vi "HFRR ADV v03.vi"() -> ()   [LabVIEW 2025] (continued)
          }
          n24 = Concatenate Strings(w97) -> (w93:string)
          n25 = local read "file path"() -> (w91:path)
          n26 = call <vilib>:"Write Characters To File.vi"("append to file? (new file:F)"=FALSE, "character string"=w93, "file path (dialog if empty)"=w91) -> ()  [unwired: 2 in, 1 out]
        }
      }
      n27 = local write "refresh flag"(FALSE ("refresh flag")) -> ()
      n28 = local write "Json End Flg"(w57) -> ()
      n29 = local write "Re-Initialise"(TRUE ("Re-Initialise")) -> ()
      n30 = local write "Upld AR 2"(TRUE ("Upld AR 2")) -> ()
      n31 = local write "Json St Flg"(w57) -> ()
      n32 = local write "FLAG 2"(0.0 ("FLAG 2")) -> ()
      n33 = local write "Lan flag"(0.0 ("Lan flag")) -> ()
      n34 = local write "Flag"(0.0 ("Flag")) -> ()
      n35 = local write "clk"(0.0 ("clk")) -> ()
      n36 = local write "COUNT"(0 ("COUNT")) -> ()
      n37 = case shown="True" "STOP" {
        frame False {
        }
        frame True {
          n38 = local write "STOP 3"(TRUE ("STOP")) -> ()
        }
      }
      n39 = local write "conststatus"(0.0 ("rpm value : 2")) -> ()
      "file path" <- path "C:/Windows/wndcm_pw_stdED hfrr.txt" ("file path")
      "FF buffer" <- dbl[] [] ("FF buffer")
    }
    frame #1 {
      n40 = Wait (ms)(milliseconds to wait=u32 1000) -> (millisecond timer value=w109:u32)
    }
    frame #2 {
      n41 = local read "Re-Initialise"() -> (w112:bool)
      n42 = case shown="True" w112 {
        frame False {
        }
        frame True {
          n43 = local write "Re-Initialise"(FALSE ("Re-Initialise")) -> ()
        }
      }
    }
  }
  n44 = local write "main tab sub"(enum32{"Page 1", "Page 2"}."Page 1" ("main tab sub")) -> ()
  n45 = local write "USERNAME"(w5) -> ()
  n46 = local write "USER ID"(w5) -> ()
  n47 = local write "Main Tab"(T1."HOME" ("Main Tab")) -> ()
  n48 = property on="Quit" class="Bool (strict)"("Value"=FALSE ("Quit")) -> (error out=w7:errorcluster)  [unwired: 2 in, 1 out]
  n49 = while {
    tunnel: w7 -> [_]
    stop <- w137 stop-if-true
    w128 = 1 ("y")
    # "New Adv Logics"
    n50 = local read "USERNAME"() -> (w134:string)
    n51 = local read "Sign In"() -> (w124:bool)
    n52 = local read "USER ID"() -> (w131:string)
    n53 = local read "Dashboard"() -> (w122:bool)
    n54 = local read "Imaging"() -> (w119:bool)
    n55 = local read "Test Setup"() -> (w123:bool)
    n56 = Wait (ms)(milliseconds to wait=u32 100) -> ()  [unwired: 1 out]
    n57 = case shown="True" w124 {
      selector: w124 -> [_ w164]
      frame False {
      }
      frame True {
        n58 = Not(x=w164) -> (.not. x?=w163:bool)
        n59 = local write "Sign In"(w163) -> ()
        n60 = local write "Main Tab"(T1."Test Setup" ("Main Tab")) -> ()
      }
    }
    n61 = call <vilib>:"Trim Whitespace.vi"("string"=w134) -> ("trimmed string"=w133:string)  [unwired: 1 in]
    n62 = call <vilib>:"Trim Whitespace.vi"("string"=w131) -> ("trimmed string"=w132:string)  [unwired: 1 in]
    n63 = case shown="True" w122 {
      selector: w122 -> [_ w158]
      frame False {
      }
      frame True {
        n64 = Not(x=w158) -> (.not. x?=w157:bool)
        n65 = local write "Dashboard"(w157) -> ()
        n66 = local write "Main Tab"(T1."Acquire" ("Main Tab")) -> ()
      }
    }
    n67 = String Length(string=w133) -> (length=w130:i32)
    n68 = String Length(string=w132) -> (length=w129:i32)
    n69 = case shown="True" w123 {
      selector: w123 -> [_ w161]
      frame False {
      }
      frame True {
        n70 = Not(x=w161) -> (.not. x?=w160:bool)
        n71 = local write "Test Setup"(w160) -> ()
        n72 = local write "Main Tab"(T1."HOME" ("Main Tab")) -> ()
      }
    }
    n73 = case shown="True" w119 {
      selector: w119 -> [_ w148]
      frame False {
      }
      frame True {
        n74 = Not(x=w148) -> (.not. x?=w147:bool)
        n75 = local write "Imaging"(w147) -> ()
        n76 = local write "Main Tab"(T1."Adv Scar" ("Main Tab")) -> ()
      }
    }
    n77 = local read "Main Tab"() -> (w135:T1)
    n78 = Greater?(x=w130, y=w128) -> (0:w127:bool)
    n79 = Greater?(x=w129, y=w128) -> (0:w126:bool)
    n80 = And(x=w127, y=w126) -> (x .and. y?=w125:bool)
    n81 = case shown="\"HOME\"" w135 {
      frame "HOME" {
        n82 = local write "main tab sub"(enum32{"Page 1", "Page 2"}."Page 1" ("main tab sub")) -> ()
      }
      frame Default {
        n83 = local write "main tab sub"(enum32{"Page 1", "Page 2"}."Page 2" ("main tab sub")) -> ()
      }
    }
    n84 = case shown="False" w125 {
      frame False {
        n85 = property on="Sign In" class="Bool (strict)"("DisabledEnum"=T11."Disabled" ("Disabled")) -> ()  [unwired: 2 in, 2 out]
      }
      frame True {
        n86 = property on="Sign In" class="Bool (strict)"("DisabledEnum"=T11."Enabled" ("Disabled")) -> ()  [unwired: 2 in, 2 out]
      }
    }
    n87 = local read "Report"() -> (w118:bool)
    n88 = local read "Button"() -> (w121:bool)
    n89 = case shown="True" w118 {
      selector: w118 -> [_ w145]
      frame False {
      }
      frame True {
        n90 = Not(x=w145) -> (.not. x?=w144:bool)
        n91 = local write "Report"(w144) -> ()
        n92 = local write "Main Tab"(T1."Adv Scar Report" ("Main Tab")) -> ()
      }
    }
    n93 = local read "Button 2"() -> (w120:bool)
    n94 = local read "Analysis"() -> (w117:bool)
    n95 = case shown="True" w121 {
      selector: w121 -> [_ w154]
      frame False {
      }
      frame True {
        n96 = Not(x=w154) -> (.not. x?=w153:bool)
        n97 = local write "Button"(w153) -> ()
        n98 = local write "Main Tab Display"(enum32{"Dashboard 1", "Dashboard 2"}."Dashboard 1" ("Main Tab Display")) -> ()
      }
    }
    n99 = case shown="True" w120 {
      selector: w120 -> [_ w152]
      frame False {
      }
      frame True {
        n100 = Not(x=w152) -> (.not. x?=w151:bool)
        n101 = local write "Button 2"(w151) -> ()
        n102 = local write "Main Tab Display"(enum32{"Dashboard 1", "Dashboard 2"}."Dashboard 2" ("Main Tab Display")) -> ()
      }
    }
    n103 = case shown="True" w117 {
      selector: w117 -> [_ w143]
      frame False {
      }
      frame True {
        n104 = Not(x=w143) -> (.not. x?=w141:bool)
        n105 = local write "Analysis"(w141) -> ()
        n106 = local write "Main Tab"(T1."Compare Files" ("Main Tab")) -> ()
      }
    }
    n107 = local read "About"() -> (w116:bool)
    n108 = case shown="True" w116 {
      selector: w116 -> [_ w140]
      frame False {
      }
      frame True {
        n109 = Not(x=w140) -> (.not. x?=w139:bool)
        n110 = local write "About"(w139) -> ()
        n111 = local write "Main Tab"(T1."About" ("Main Tab")) -> ()
      }
    }
    n112 = local read "Quit"() -> (w137:bool)
  }
  n113 = while {
    stop <- w173 stop-if-true
    n114 = local read "Image Path"() -> (w171:path)
    n115 = local read "Print 3"() -> (w175:bool)
    n116 = Equal?(x=w171, y=path "") -> (x = y?=w170:bool)
    n117 = Not(x=w170) -> (.not. x?=w169:bool)
    n118 = property on="Print 3" class="Bool (strict)"("Visible"=w169) -> ()  [unwired: 2 in, 2 out]
    n119 = case shown="True" w175 {
      frame False {
        n120 = local write "Rd"(TRUE ("Boolean 7")) -> ()
      }
      frame True {
        n121 = flat-sequence {
          tunnel: [w215] -> w183
          tunnel: [w202] -> w181
          tunnel: [w212] -> w177
          tunnel: w183 -> [w224]
          tunnel: [w224] -> w182
          tunnel: w181 -> [w223]
          tunnel: [w223] -> w180
          tunnel: [w221] -> w179
          tunnel: [w220] -> w178
          tunnel: w177 -> [w220]
          tunnel: w182 -> [w226]
          tunnel: w180 -> [w227]
          tunnel: w179 -> [_]
          tunnel: w178 -> [w225]
          frame #0 {
            n122 = case shown="True" "Rd" {
              frame False {
              }
              frame True {
                n123 = while {
                  tunnel: "abcdefABCDEF" ("string 2") -> [w194]
                  shift-right: [w192] -> w186
                  shift-left: "" -> [w191]
                  i -> [w201]
                  stop <- w200 stop-if-true
                  n124 = Random Number (0-1)() -> (number: 0 to 1=w195:dbl)
                  n125 = Multiply(x=w195, y=62.0) -> (x*y=w197:dbl)
                  n126 = Decrement(x="Length 2") -> (x-1=w190:i16)
                  n127 = To Word Integer(number=w197) -> (16bit integer=w198:i16)
                  n128 = String Subset(string=w194, offset (0)=w198, length (rest)=1 ("length (rest)")) -> (substring=w193:string)
                  n129 = Greater Or Equal?(x=w201, y=w190) -> (x >= y?=w200:bool)
                  n130 = Concatenate Strings(w193, w191) -> (w192:string)
                }
                "String 10" <- w186
                n131 = local write "Rd"(FALSE ("Boolean 7")) -> ()
              }
            }
          }
          frame #1 {
            w213 = "_resized.jpg" ("command line")
            (unwired) ".jpg -resize 320x240 " ("string")
            (unwired) "Choose an Image File" ("prompt")
            # "-resize 1798x425"
            n132 = local read "Image Path"() -> (w207:path)
            n133 = Strip Path(path=w207) -> (stripped path=w202:path, name=w203:string)
            n134 = Match Pattern(string=w203, regular expression=".jpg") -> (before substring=→"before substring 2":string, after substring=→"after substring":string)  [unwired: 1 in, 2 out]
            n135 = Match Pattern(string=w203, regular expression="\\") -> (before substring=w209:string)  [unwired: 1 in, 3 out]
            n136 = Match Pattern(string=w209, regular expression=".jpg") -> (before substring=w208:string)  [unwired: 1 in, 3 out]
            n137 = Concatenate Strings("cmd /c convert " ("string"), w208, ".jpg -resize 320x240  " ("command line"), w208, w213) -> (w216:string)
            n138 = call <vilib>:"System Exec.vi"("run minimized? (F)"=TRUE, "wait until completion? (T)"=TRUE, "working directory"=w202, "command line"=w216) -> ("error out"=w215:errorcluster)  [unwired: 4 in, 3 out]
            "error out 2" <- w215
            n139 = Concatenate Strings(w208, w213) -> (w212:string)
          }
          frame #2 {
            n140 = Wait (ms)(milliseconds to wait=u32 2000 ("millisecond timer value")) -> (millisecond timer value=w221:u32)
          }
          frame #3 {
            n141 = case shown="No Error" w226 {
              tunnel: w227 -> [w230 _]
              tunnel: w225 -> [w228 _]
              frame No Error {
                (unwired) ".jpg" ("string")
                n142 = Path To String(path=w230) -> (string=w234:string)
                n143 = Concatenate Strings(w234, "\\" ("string"), w228) -> (w233:string)
                n144 = String To Path(string=w233) -> (path=w232:path)
                n145 = call <vilib>:"Read JPEG File.vi"("path to JPEG file"=w232) -> ("image data"=w236:T8)  [unwired: 8 in, 2 out]
                "image data" <- w236
                n146 = local write "Print 3"(FALSE ("Print 2")) -> ()
                n147 = call <vilib>:"Draw Flattened Pixmap.vi"("image data"=w236) -> ("new picture"=→"new picture":picture)  [unwired: 8 in]
              }
              frame Error {
              }
            }
          }
        }
      }
    }
    n148 = Wait (ms)(milliseconds to wait=u32 20 ("millisecond timer value")) -> ()  [unwired: 1 out]
    n149 = local read "EXIT"() -> (w173:bool)
  }
  n150 = case shown="True" "Case Constant\n(See Context Help) 7" {
    tunnel: [_ w238] -> w25
    tunnel: w23 -> [_ w237]
    frame False {
    }
    frame True {
      n151 = while {
        tunnel: w237 -> [_]
        tunnel: [w240] -> w238
        tunnel: [w239] -> _
        i -> [w239]
        stop <- w240 stop-if-true
        w256 = u16 10 items=["1.0"=10, "1.5"=15, "2.0"=20] ("stop bits (10: 1 bit)")
        n152 = Wait (ms)(milliseconds to wait=u32 10) -> ()  [unwired: 1 out]
        n153 = call-poly "VISA Configure Serial Port"("VISA resource name"=refnum<visa-resource-name> "ASRL1::INSTR" ("COM PORT"), "timeout (10sec)"=u32 10, "baud rate (9600)"=u32 57600, "data bits (8)"=u16 8, "stop bits (10: 1 bit)"=w256) -> ("VISA resource name out"=w242:refnum<visa-resource-name>, "error out"=w251:errorcluster)  [unwired: 9 in]
        n154 = VISA Read(VISA resource name=w242, byte count=u32 2 ("byte count (0)")) -> (read buffer=w250:string)  [unwired: 1 in, 3 out]
        n155 = String Subset(string=w250, offset (0)=0, length (rest)=2 ("length (rest)")) -> (substring=w249:string)
        n156 = Match Pattern(string=w249, regular expression="<>") -> (offset past match=w246:i32)  [unwired: 1 in, 3 out]
        n157 = Greater Or Equal?(x=w246, y=0) -> (x >= y?=w241:bool)
        n158 = case shown="True" w241 {
          tunnel: w242 -> [_ w260]
          tunnel: w251 -> [_ w259]
          frame False {
          }
          frame True {
            n159 = VISA Read(VISA resource name=w260, byte count=u32 32 ("byte count (0)"), error in (no error)=w259) -> (read buffer=w258:string)  [unwired: 3 out]
            n160 = String Subset(string=w258, offset (0)=0, length (rest)=8 ("length (rest)")) -> (substring=w262:string)
            n161 = String Subset(string=w258, offset (0)=8, length (rest)=8 ("length (rest)")) -> (substring=w263:string)
            n162 = Decimal String To Number(string=w263) -> (number=w270:i32)  [unwired: 2 in, 1 out]
            n163 = Decimal String To Number(string=w262) -> (number=w266:i32)  [unwired: 2 in, 1 out]
            n164 = Divide(x=w270, y=10000) -> ()  [unwired: 1 out]
            n165 = Divide(x=w266, y=1000000) -> ()  [unwired: 1 out]
          }
        }
        n166 = local read "EXIT"() -> (w240:bool)
      }
    }
  }
  n167 = local write "Err Count"(0 ("Err Count")) -> ()
  n168 = local write "FRICVALZ"(0.0 ("FRICVALZ")) -> ()
  n169 = Tick Count (ms)() -> (millisecond timer value=w43:u32)
  n170 = while {
    shift-right: [w287] -> w19
    shift-left: _ -> [w277]
    shift-right: [w286] -> w18
    shift-left: errorcluster {"status"=FALSE, "code"=0, "source"="Init"} ("error out") -> [w279]
    tunnel: [w284] -> w33
    tunnel: [w285] -> _
    tunnel: w23 -> [_]
    i -> [w285]
    stop <- w284 stop-if-true
    n171 = local read "Re-Initialise"() -> (w272:bool)
    n172 = Unbundle(w279) -> ("status"=→"Port 4":bool)  [unwired: 2 out]
    n173 = flat-sequence {
      tunnel: w279 -> [w291]
      tunnel: [w291] -> w275
      frame #0 {
        n174 = Wait (ms)(milliseconds to wait=u32 50) -> ()  [unwired: 1 out]
      }
    }
    n175 = local read "Com Port 2"() -> (w278:refnum<visa-resource-name>)
    n176 = Not Equal?(x=w278, y=w277) -> (x != y?=w276:bool)
    n177 = Or(x=w276, y=w272) -> (x .or. y?=w273:bool)
    n178 = case shown="True" w273 {
      tunnel: [w288 errorcluster {"status"=TRUE, "code"=0, "source"="Init"} ("error out")] -> w274
      tunnel: w275 -> [w288 _]
      frame False {
      }
      frame True {
      }
    }
    n179 = case shown="Error" w274 {
      selector: w274 -> [w294 w448]
      tunnel: [w296 w453] -> w287
      tunnel: [w295 w446] -> w286
      tunnel: w277 -> [w298 w451]
      tunnel: [w297 _] -> _
      frame No Error {
        n180 = stacked-sequence {
          tunnel: w298 -> [w322 _]
          tunnel: w294 -> [w321 _]
          tunnel: [w308 _] -> w297
          tunnel: [w307 _] -> w296
          tunnel: [w306 _] -> w295
          frame #0 {
            n181 = property class="Instr"(reference=w322, error in=w321) -> (reference out=w305:refnum<visa-resource-name>, error out=w320:errorcluster, "Serial Settings:Number of Bytes at Serial Port"=w301:u32)
            "Port 2" <- w301
            n182 = Greater?(x=w301, y=u32 23) -> (0:w303:bool)
            n183 = Not(x=w303) -> ()  [unwired: 1 out]
            n184 = call "Elapsed Time10"("Time Target (s)"=2.0, "Reset"=w303, "Auto Reset"=FALSE) -> ("Time has Elapsed"=→"Port 2a":bool)  [unwired: 9 in, 7 out]
            n185 = case shown="True" w303 {
              tunnel: w305 -> [w337 w362]
              tunnel: w320 -> [w336 w363]
              tunnel: [w336 w365] -> w316
              tunnel: [w337 w364] -> w317
              frame False {
              }
              frame True {
                # "Out as Volts"
                n186 = local read "Residual Due"() -> (w361:string)
                n187 = while {
                  tunnel: [w405] -> w365
                  tunnel: [w404] -> w364
                  tunnel: w363 -> [w403]
                  tunnel: w362 -> [w402]
                  tunnel: [w399] -> _
                  shift-right: [w397] -> w360
                  shift-left: w361 -> [w396]
                  i -> [w399]
                  stop <- w400 stop-if-true
                  n188 = property class="Instr"(reference=w402, error in=w403) -> (reference out=w407:refnum<visa-resource-name>, error out=w406:errorcluster, "Serial Settings:Number of Bytes at Serial Port"=w398:u32)
                  n189 = Greater?(x=w398, y=u32 8) -> (0:w400:bool)
                  n190 = VISA Read(VISA resource name=w407, byte count=w398, error in (no error)=w406) -> (VISA resource name out=w404:refnum<visa-resource-name>, read buffer=w395:string, error out=w405:errorcluster)  [unwired: 1 out]
                  n191 = Concatenate Strings(w396, w395) -> (w397:string)
                }
                n192 = while {
                  shift-right: [w388] -> w344
                  shift-left: w360 -> [w393]
                  tunnel: [w387] -> w356 mode=indexing
                  tunnel: [w386] -> _
                  i -> [w386]
                  stop <- w390 stop-if-true
                  n193 = Match Pattern(string=w393, regular expression="*") -> (after substring=w391:string)  [unwired: 1 in, 3 out]
                  n194 = Match Pattern(string=w391, regular expression="&") -> (before substring=w387:string, after substring=w388:string, offset past match=w389:i32)  [unwired: 1 in, 1 out]
                  n195 = Less Than 0?(x=w389) -> (x < 0?=w390:bool)
                }
                n196 = local write "Residual Due"(w344) -> ()
                n197 = Array Size(array=w356) -> (size(s)=w359:i32)
                n198 = Decrement(x=w359) -> (x-1=w357:i32)
                n199 = Delete From Array(array=w356, length=1, index=w357) -> (array with subset deleted=w355:string[])  [unwired: 1 out]
                n200 = Array Size(array=w355) -> (size(s)=w343:i32)
                n201 = Decrement(x=w343) -> (x-1=w342:i32)
                n202 = while {
                  tunnel: w355 -> [w374] mode=indexing
                  tunnel: w342 -> [w373]
                  tunnel: [w371] -> w350 mode=indexing
                  tunnel: [w370] -> w349 mode=indexing
                  tunnel: [w369] -> w348 mode=indexing
                  tunnel: [w368] -> w347 mode=indexing
                  tunnel: [w367] -> w345 mode=indexing
                  tunnel: [w366] -> _
                  i -> [w366]
                  stop <- w372 stop-if-true
                  w383 = u32 0 ("length (rest)")
                  w382 = ";" ("regular expression")
                  n203 = Match Pattern(string=w374, regular expression=w382) -> (before substring=w375:string, after substring=w376:string)  [unwired: 1 in, 2 out]
                  n204 = Match Pattern(string=w376, regular expression=w382) -> (before substring=w379:string, after substring=w377:string)  [unwired: 1 in, 2 out]
                  n205 = Less Or Equal?(x=w373, y=w366) -> (x <= y?=w372:bool)
                  n206 = Match Pattern(string=w377, regular expression=w382) -> (before substring=w380:string, after substring=w378:string)  [unwired: 1 in, 2 out]
                  n207 = Match Pattern(string=w378, regular expression=w382) -> (before substring=w381:string, after substring=w385:string)  [unwired: 1 in, 2 out]
                  n208 = Decimal String To Number(string=w375, default (0L)=w383) -> (number=w371:u32)  [unwired: 1 in, 1 out]
                  n209 = Decimal String To Number(string=w379, default (0L)=w383) -> (number=w370:u32)  [unwired: 1 in, 1 out]
                  n210 = Decimal String To Number(string=w380, default (0L)=w383) -> (number=w369:u32)  [unwired: 1 in, 1 out]
                  n211 = Decimal String To Number(string=w381, default (0L)=w383) -> (number=w368:u32)  [unwired: 1 in, 1 out]
                  n212 = Decimal String To Number(string=w385, default (0L)=u8 0 ("length (rest)")) -> (number=w367:u8)  [unwired: 1 in, 1 out]
                }
                "Din" <- w345
                n213 = Bundle(w350, w349, w348, w347) -> (w352:cluster{u32[], u32[], u32[], u32[]})  [unwired: 1 in]
                n214 = Divide(x=w352, y=4095 ("length (rest)")) -> (x/y=w354:cluster{dbl[], dbl[], dbl[], dbl[]})
                n215 = Multiply(x=w354, y=sgl 3.32 ("Numeric")) -> (x*y=w346:cluster{dbl[], dbl[], dbl[], dbl[]})
                n216 = Unbundle(w346) -> (→"ECR":dbl[], →"Rtemp":dbl[], →"Air temp":dbl[], →"Ch3 2":dbl[])
              }
            }
            n217 = local read "Due Com"() -> (w309:string[])
            n218 = Delete From Array(array=w309, length=1, index=0) -> (deleted portion=w312:string[], array with subset deleted=w313:string[])
            n219 = local write "Due Com"(w313) -> ()
            n220 = Index Array(array=w312, index=0) -> (element=w310:string)
            n221 = Not Equal?(x=w310, y="") -> (x != y?=w318:bool)
            n222 = case shown="True" w318 {
              tunnel: w317 -> [w324 w329]
              tunnel: [w324 w333] -> w307
              tunnel: w316 -> [w323 w328]
              tunnel: [w323 w331] -> w306
              tunnel: w310 -> [_ w327]
              tunnel: [_ w330] -> _
              frame False {
                # "DATA  WRITE LOOP"
              }
              frame True {
                n223 = Concatenate Strings(w327, "\r\n") -> (w326:string)
                n224 = VISA Write(VISA resource name=w329, write buffer=w326, error in (no error)=w328) -> (VISA resource name out=w333:refnum<visa-resource-name>, return count=w330:u32, error out=w332:errorcluster)
                n225 = flat-sequence {
                  tunnel: w332 -> [w334]
                  tunnel: [w334] -> w331
                  frame #0 {
                    n226 = Wait (ms)(milliseconds to wait=u32 5) -> ()  [unwired: 1 out]
                  }
                }
              }
            }
            n227 = Array Size(array=w309) -> (size(s)=w308:i32)
          }
          frame #1 {
            w416 = 10 ("y")
            w421 = 10 ("y")
            n228 = local read "Rtemp"() -> (w409:dbl[])
            n229 = for {
              tunnel: w409 -> [w433] mode=indexing
              shift-right: [w434] -> w417
              shift-left: dbl[] [] ("temp buf 2") -> [w435]
              n230 = Equal To 0?(x=w433) -> (x = 0?=w437:bool)
              n231 = Build Array (concatenate)(w435, w433) -> (w436:dbl[])
              n232 = Select(t=w435, s=w437, f=w436) -> (s? t:f=w434:dbl[])
            }
            n233 = local read "temp buf"() -> (w418:dbl[])
            n234 = Insert Into Array(array=w417, index=0, new element=w418) -> (w423:dbl[])
            n235 = Array Size(array=w423) -> (size(s)=w422:i32)
            n236 = Greater?(x=w422, y=w421) -> (0:w424:bool)
            n237 = case shown="True" w424 {
              tunnel: w423 -> [w438 w444]
              tunnel: w422 -> [_ w442]
              tunnel: w421 -> [_ w441]
              tunnel: [w438 w439] -> w420
              frame False {
              }
              frame True {
                n238 = Subtract(x=w442, y=w441) -> (x-y=w440:i32)
                n239 = Delete From Array(array=w444, length=w440, index=0) -> (array with subset deleted=w439:dbl[])  [unwired: 1 out]
              }
            }
            "temp buf" <- w420
            n240 = local read "ecr buf"() -> (w410:dbl[])
            n241 = local read "ECR"() -> (w408:dbl[])
            n242 = Insert Into Array(array=w408, index=0, new element=w410) -> (w414:dbl[])
            n243 = Array Size(array=w414) -> (size(s)=w415:i32)
            n244 = Greater?(x=w415, y=w416) -> (0:w413:bool)
            n245 = case shown="True" w413 {
              tunnel: w414 -> [w426 w432]
              tunnel: w415 -> [_ w430]
              tunnel: w416 -> [_ w429]
              tunnel: [w426 w427] -> w411
              frame False {
              }
              frame True {
                n246 = Subtract(x=w430, y=w429) -> (x-y=w428:i32)
                n247 = Delete From Array(array=w432, length=w428, index=0) -> (array with subset deleted=w427:dbl[])  [unwired: 1 out]
              }
            }
            "ecr buf" <- w411
          }
        }
      }
      frame Error {
        w459 = u16 0 items=["None", "XON/XOFF", "RTS/CTS", "XON/XOFF & RTS/CTS", "DTR/DSR", "XON/XOFF & DTR/DSR"] ("flow control (0:none)  2")
        w457 = u16 10 items=["1.0"=10, "1.5"=15, "2.0"=20] ("stop bits 2")
        w455 = u16 0 items=["None", "Odd", "Even", "Mark", "Space"] ("parity 2")
        w456 = u32 10000  # timeout (10sec)
        n248 = VISA Clear(VISA resource name=w451, error in (no error)=w448) -> (VISA resource name out=w450:refnum<visa-resource-name>, error out=w449:errorcluster)
        n249 = VISA Close(VISA resource name=w450, error in (no error)=w449) -> (error out=w452:errorcluster)
        n250 = local read "Com Port 2"() -> (w445:refnum<visa-resource-name>)
        "visa due" <- w445
        n251 = call <vilib>:"Clear Errors.vi"("error in (no error)"=w452) -> ()  [unwired: 5 in, 2 out]
        n252 = call-poly "VISA Configure Serial Port"("VISA resource name"=w445, "timeout (10sec)"=w456, "baud rate (9600)"=u32 250000 ("baud rate  2"), "data bits (8)"=u16 8 ("data bits  2"), "parity (0:none)"=w455, "stop bits (10: 1 bit)"=w457, "flow control (0:none)"=w459) -> ("VISA resource name out"=w460:refnum<visa-resource-name>, "error out"=w461:errorcluster)  [unwired: 7 in]
        n253 = flat-sequence {
          tunnel: w460 -> [w463]
          tunnel: w461 -> [w462]
          tunnel: [w463] -> w453
          tunnel: [w462] -> w446
          frame #0 {
            n254 = Wait (ms)(milliseconds to wait=u32 50) -> ()  [unwired: 1 out]
          }
        }
        "Residual Due" <- ""
        "Port 2 Error" <- w446
      }
    }
    n255 = local read "Port 2a"() -> (w280:bool)
    n256 = local read "Port 4"() -> (w281:bool)
    n257 = Or(x=w281, y=w280) -> (x .or. y?=w283:bool)
    n258 = case shown="True" w283 {
      frame False {
        w292 = FALSE ("Visible")
        n259 = property on="Port 2a" class="Bool (strict)"("Visible"=w292) -> ()  [unwired: 2 in, 2 out]
        n260 = property on="Port 4" class="Bool (strict)"("Visible"=w292) -> ()  [unwired: 2 in, 2 out]
      }
      frame True {
        w293 = TRUE ("Visible")
        n261 = property on="Port 2a" class="Bool (strict)"("Visible"=w293) -> ()  [unwired: 2 in, 2 out]
        n262 = property on="Port 4" class="Bool (strict)"("Visible"=w293) -> ()  [unwired: 2 in, 2 out]
      }
    }
    n263 = local read "EXIT"() -> (w284:bool)
    "Error Due" <- w279
  }
  n264 = while {
    shift-right: [w482] -> w47
    shift-left: _ -> [w470]
    shift-right: [w481] -> w46
    shift-left: errorcluster {"status"=TRUE, "code"=0, "source"="Init"} ("error IO") -> [w472]
    shift-right: [w479] -> _
    shift-left: w43 -> [w480]
    tunnel: w23 -> [_]
    tunnel: [w478] -> w34
    tunnel: [w477] -> _
    i -> [w477]
    stop <- w478 stop-if-true
    n265 = local read "Com Port 1"() -> (w471:refnum<visa-resource-name>)
    n266 = flat-sequence {
      tunnel: [w485] -> w468
      tunnel: w472 -> [w485]
      frame #0 {
        n267 = Wait (ms)(milliseconds to wait=u32 200) -> ()  [unwired: 1 out]
      }
    }
    n268 = local read "Re-Initialise"() -> (w465:bool)
    n269 = Not Equal?(x=w471, y=w470) -> (x != y?=w469:bool)
    n270 = Or(x=w469, y=w465) -> (x .or. y?=w466:bool)
    n271 = Unbundle(w472) -> ("status"=→"Port 3":bool)  [unwired: 2 out]
    n272 = case shown="True" w466 {
      tunnel: [w483 errorcluster {"status"=TRUE, "code"=0, "source"="Init"} ("error out")] -> w467
      tunnel: w468 -> [w483 _]
      frame False {
      }
      frame True {
      }
    }
    n273 = case shown="No Error" w467 {
      selector: w467 -> [w489 w815]
      tunnel: [w494 w820] -> w482
      tunnel: [w493 w812] -> w481
      tunnel: w470 -> [w492 w818]
      tunnel: w480 -> [w491 w817]
      tunnel: [w490 w817] -> w479
      frame No Error {
        n274 = stacked-sequence {
          tunnel: [w504 _ _ _ _ _] -> w494
          tunnel: [w503 _ _ _ _ _] -> w493
          tunnel: w492 -> [w499 _ _ _ _ _]
          tunnel: w489 -> [w498 _ _ _ _ _]
          tunnel: w491 -> [_ w612 _ _ _ _]
          tunnel: [_ w611 _ _ _ _] -> w490
          tunnel: [_ w583 _ _ _ _] -> _
          frame #0 {
            n275 = property class="Instr"(reference=w499, error in=w498) -> (reference out=w501:refnum<visa-resource-name>, error out=w502:errorcluster, "Serial Settings:Number of Bytes at Serial Port"=w495:u32)
            "Sps 3" <- w495
            "Port 1" <- w495
            n276 = Greater?(x=w495, y=u32 5) -> (0:w497:bool)
            n277 = Not(x=w497) -> (.not. x?=→"Port 1a":bool)
            n278 = case shown="True" w497 {
              tunnel: w501 -> [w506 w527]
              tunnel: w502 -> [w505 w528]
              tunnel: [w505 w530] -> w503
              tunnel: [w506 w529] -> w504
              frame False {
              }
              frame True {
                # "Out as Volts"
                n279 = local read "Residual Uno"() -> (w521:string)
                n280 = while {
                  tunnel: [w567] -> w530
                  tunnel: [w566] -> w529
                  tunnel: w528 -> [w565]
                  tunnel: w527 -> [w564]
                  tunnel: [w561] -> _
                  shift-right: [w557] -> w509
                  shift-left: w521 -> [w559]
                  i -> [w561]
                  stop <- w562 stop-if-true
                  n281 = property class="Instr"(reference=w564, error in=w565) -> (reference out=w569:refnum<visa-resource-name>, error out=w568:errorcluster, "Serial Settings:Number of Bytes at Serial Port"=w560:u32)
                  n282 = Greater?(x=w560, y=u32 30) -> (0:w562:bool)
                  n283 = VISA Read(VISA resource name=w569, byte count=w560, error in (no error)=w568) -> (VISA resource name out=w566:refnum<visa-resource-name>, read buffer=w558:string, error out=w567:errorcluster)  [unwired: 1 out]
                  n284 = Concatenate Strings(w559, w558) -> (w557:string)
                }
                "UnoRead" <- w509
                n285 = while {
                  shift-right: [w543] -> w520
                  shift-left: w509 -> [w549]
                  tunnel: [w542] -> w516 mode=indexing
                  tunnel: [w544] -> _
                  i -> [w544]
                  stop <- w546 stop-if-true
                  n286 = Match Pattern(string=w549, regular expression="*") -> (after substring=w547:string)  [unwired: 1 in, 3 out]
                  n287 = Match Pattern(string=w547, regular expression="&") -> (before substring=w542:string, after substring=w543:string, offset past match=w545:i32)  [unwired: 1 in, 1 out]
                  n288 = Less Than 0?(x=w545) -> (x < 0?=w546:bool)
                }
                n289 = local write "Residual Uno"(w520) -> ()
                n290 = Array Size(array=w516) -> (size(s)=w517:i32)
                n291 = Decrement(x=w517) -> (x-1=w519:i32)
                n292 = Delete From Array(array=w516, length=1, index=w519) -> (array with subset deleted=w514:string[])  [unwired: 1 out]
                n293 = Array Size(array=w514) -> (size(s)=w513:i32)
                n294 = Decrement(x=w513) -> (x-1=w512:i32)
                n295 = while {
                  tunnel: [w541] -> w525 mode=indexing
                  tunnel: [w540] -> w524 mode=indexing
                  tunnel: w514 -> [w534] mode=indexing
                  tunnel: w512 -> [w533]
                  tunnel: [w531] -> _
                  i -> [w531]
                  stop <- w532 stop-if-true
                  w535 = 0 ("length (rest)")
                  w537 = ";" ("regular expression")
                  n296 = Match Pattern(string=w534, regular expression=w537) -> (before substring=w539:string, after substring=w538:string)  [unwired: 1 in, 2 out]
                  n297 = Match Pattern(string=w538, regular expression=w537) -> (before substring=w536:string)  [unwired: 1 in, 3 out]
                  n298 = Less Or Equal?(x=w533, y=w531) -> (x <= y?=w532:bool)
                  n299 = Decimal String To Number(string=w539, default (0L)=w535) -> (number=w541:i32)  [unwired: 1 in, 1 out]
                  n300 = Decimal String To Number(string=w536, default (0L)=w535) -> (number=w540:i32)  [unwired: 1 in, 1 out]
                }
                n301 = Bundle(w525, w524) -> (w515:cluster{i32[], i32[]})  [unwired: 1 in]
                n302 = case shown="0, Default" "ADC Res" {
                  tunnel: [w552 w554] -> w508
                  frame 0, Default {
                    n303 = Divide(x=65535 ("length (rest)"), y=2 ("length (rest)")) -> (x/y=w552:dbl)
                  }
                  frame 1 {
                    n304 = Divide(x=16777216 ("length (rest)"), y=2 ("length (rest)")) -> (x/y=w554:dbl)
                  }
                }
                n305 = Divide(x=w515, y=w508) -> (x/y=w526:cluster{dbl[], dbl[]})
                n306 = Multiply(x=w526, y=sgl 5.03 ("Numeric")) -> (x*y=w523:cluster{dbl[], dbl[]})
                n307 = Unbundle(w523) -> (→"Ch1":dbl[], →"Ch0":dbl[])
              }
            }
          }
          frame #1 {
            n308 = local read "Ch1"() -> (w594:dbl[])
            n309 = call-poly <vilib>:"Mean.vi"("X"=w594) -> ("mean"=w595:dbl)  [unwired: 1 out]
            "Slide 3" <- w595
            n310 = call <vilib>:"Mean PtByPt.vi"("x"=w595, "sample length"=10, "initialize"="Reset 2") -> ("mean"=→"Mean Pos Fil 2":dbl)  [unwired: 1 in, 1 out]
            n311 = case shown="True" "Zero 2" {
              tunnel: w594 -> [_ w624]
              frame False {
              }
              frame True {
                n312 = call-poly <vilib>:"Mean.vi"("X"=w624) -> ("mean"=→"zOff 2":dbl)  [unwired: 1 out]
                n313 = local write "Zero 2"(FALSE ("Zero")) -> ()
              }
            }
            n314 = Tick Count (ms)() -> (millisecond timer value=w611:u32)
            n315 = local read "zOff 2"() -> (w604:dbl)
            n316 = Subtract(x=w611, y=w612) -> (x-y=w610:u32)
            n317 = Subtract(x=w594, y=w604) -> (x-y=w600:dbl[])
            n318 = Divide(x=w610, y=u32 1000 ("x")) -> (x/y=w608:dbl)
            n319 = Multiply(x=w600, y=1.0 ("PG Oth")) -> (x*y=w586:dbl[])
            n320 = Divide(x=w586, y=1) -> (x/y=w585:dbl[])
            "Fric Val" <- w585
            n321 = local read "FF buffer"() -> (w591:dbl[])
            n322 = call-poly <vilib>:"Mean.vi"("X"=w585) -> ("mean"=w599:dbl)  [unwired: 1 out]
            n323 = Array Size(array=w591) -> (size(s)=w593:i32)
            n324 = case shown="True" "DC corr 2" {
              tunnel: w585 -> [w627 w630]
              tunnel: [w627 w629] -> w592
              tunnel: w599 -> [_ w628]
              frame False {
              }
              frame True {
                n325 = Subtract(x=w630, y=w628) -> (x-y=w629:dbl[])
              }
            }
            n326 = Insert Into Array(array=w591, index=w593, new element=w585) -> (w588:dbl[])
            n327 = Array Size(array=w592) -> (size(s)=w607:i32)
            n328 = Array Size(array=w588) -> (size(s)=w587:i32)
            n329 = Divide(x=w607, y=w608) -> (x/y=w603:dbl)
            "Sps 2" <- w603
            n330 = Greater?(x=w587, y=1000) -> (0:w589:bool)
            n331 = Reciprocal(x=w603) -> (1/x=w601:dbl)
            "dt" <- w601
            n332 = case shown="True" w589 {
              tunnel: [w617 w620] -> w576
              tunnel: w588 -> [w617 w623]
              tunnel: w587 -> [_ w622]
              frame False {
              }
              frame True {
                n333 = Subtract(x=w622, y=1000) -> (x-y=w618:i32)
                n334 = Delete From Array(array=w623, length=w618, index=0) -> (array with subset deleted=w620:dbl[])  [unwired: 1 out]
              }
            }
            n335 = Bundle By Name("Y"=w592, "dt"=w601, "t0"=timestamp(0 s since 1904-01-01)) -> (w571:waveform(dbl))  [unwired: 1 in]
            n336 = local read "FRIC. FORCE :"() -> (w573:dbl)
            n337 = call "Elapsed Time5"("Time Target (s)"="check time s", "Reset"="Reset 3") -> ("Time has Elapsed"=w578:bool)  [unwired: 10 in, 7 out]
            n338 = Multiply(x=w573, y=21.1986) -> (x*y=w572:dbl)
            n339 = Multiply(x=w572, y=w571) -> (x*y=→"FF_Wfm":waveform(dbl))
            n340 = Negate(x=w576) -> (-x=w575:dbl[])
            n341 = local write "FF buffer"(w576) -> ()
            n342 = Array Max & Min(array=w575) -> (max value=w583:dbl)  [unwired: 3 out]
            n343 = Greater Or Equal?(x=w583, y="Threshold value") -> (x >= y?=w579:bool)
            n344 = And(x=w579, y=w578) -> (x .and. y?=w577:bool)
            n345 = case shown="True" w577 {
              frame False {
                n346 = local write "Reset 3"(FALSE ("Reset 3")) -> ()
              }
              frame True {
                n347 = local write "save dpt"(TRUE ("save dpt")) -> ()
                n348 = local write "Reset 3"(TRUE ("Reset 3")) -> ()
              }
            }
          }
          frame #2 {
            n349 = local read "FF buffer"() -> (w637:dbl[])
            n350 = Array Max & Min(array=w637) -> (max value=w632:dbl, min value=w633:dbl)  [unwired: 2 out]
            n351 = Multiply(x=1.0 ("y 2"), y="Threshold") -> ()  [unwired: 1 out]
            n352 = Subtract(x=w632, y=w633) -> (x-y=w634:dbl)
            n353 = Greater?(x=w634, y="Threshold") -> (0:w631:bool)
            n354 = case shown="True" w631 {
              tunnel: w637 -> [_ w644]
              tunnel: [_ w642] -> _
              frame False {
              }
              frame True {
                w643 = 1.0 ("y")
                n355 = Delete From Array(array=w644, length=100, index=0) -> (deleted portion=w649:dbl[])  [unwired: 1 out]
                n356 = local read "FRIC. FORCE :"() -> (w642:dbl)
                n357 = call-poly <vilib>:"Mean.vi"("X"=w649) -> ("mean"=w648:dbl)  [unwired: 1 out]
                n358 = Subtract(x=w644, y=w648) -> (x-y=w647:dbl[])
                n359 = Multiply(x=w643, y=w643) -> (x*y=w645:dbl)
                n360 = Multiply(x=w647, y=w645) -> (x*y=w646:dbl[])
                "FF cal val" <- w646
                n361 = Array Max & Min(array=w646) -> (max value=w639:dbl, min value=w638:dbl)  [unwired: 2 out]
                n362 = Array Size(array=w646) -> (size(s)=w640:i32)
                n363 = property on="FF Calibration g" class="WFGraph (strict)"("X Scale.Range:Minimum"=0.0 ("y"), "X Scale.Range:Maximum"=w640, "Y Scale.Range:Minimum"=w639, "Y Scale.Range:Maximum"=w638) -> ()  [unwired: 2 in, 2 out]
              }
            }
          }
          frame #3 {
            # "5"
            n364 = local read "Ch0"() -> (w667:dbl[])
            n365 = local read "DISPLACEMENT :"() -> (w737:dbl)
            n366 = local read "zOff 3"() -> (w740:dbl)
            n367 = Add(x=w667, y="Offset") -> (x+y=w666:dbl[])
            n368 = Subtract(x=w667, y=w740) -> (x-y=w724:dbl[])
            n369 = Multiply(x=w737, y=1.0) -> (x*y=w654:dbl)
            n370 = Multiply(x=w666, y="Gain") -> (x*y=w661:dbl[])
            "Voltage LVDT Acq" <- w661
            "gLVDTraw" <- w661
            n371 = case shown="True" "Zero 3" {
              tunnel: w667 -> [_ w755]
              frame False {
              }
              frame True {
                n372 = call-poly <vilib>:"Mean.vi"("X"=w755) -> ("mean"=→"zOff 3":dbl)  [unwired: 1 out]
                n373 = local write "Zero 3"(FALSE ("Zero")) -> ()
              }
            }
            n374 = Multiply(x=w654, y="DISPLACEMENT : 2") -> (x*y=w721:dbl)
            n375 = call-poly <vilib>:"Mean.vi"("X"=w661) -> ("mean"=w660:dbl)  [unwired: 1 out]
            n376 = Array Max & Min(array=w661) -> (max value=w665:dbl, min value=w664:dbl)  [unwired: 2 out]
            n377 = Multiply(x=w724, y=w654) -> (x*y=w736:dbl[])
            "ABS DP" <- w736
            n378 = Multiply(x=w724, y=w721) -> (x*y=w723:dbl[])
            n379 = local read "Standard Slip Gauge (mm)"() -> (w722:dbl)
            n380 = Subtract(x=w665, y=w664) -> (x-y=→"Pk-Pk":dbl)
            n381 = call-poly <vilib>:"Mean.vi"("X"=w736) -> ("mean"=w726:dbl)  [unwired: 1 out]
            n382 = call-poly <vilib>:"Mean.vi"("X"=w723) -> ("mean"=w653:dbl)  [unwired: 1 out]
            "Disp (mm)" <- w653
            "software msrnt" <- w653
            n383 = Subtract(x=w660, y="LvdtOff") -> (x-y=w659:dbl)
            n384 = case shown="True" "DC correction" {
              tunnel: w736 -> [w758 w761]
              tunnel: [w758 w760] -> w673
              tunnel: w726 -> [_ w759]
              frame False {
              }
              frame True {
                n385 = Subtract(x=w761, y=w759) -> (x-y=w760:dbl[])
              }
            }
            n386 = Threshold 1D Array(2:0.0 ("threshold y"), 3:w673) -> (0:w690:dbl)  [unwired: 1 in]
            n387 = Divide(x=w653, y=w722) -> (x/y=w720:dbl)
            n388 = Multiply(x=w720, y=w721) -> (x*y=→"DISPLACEMENT : 3":dbl)
            n389 = Equal To 0?(x=w690) -> (x = 0?=w691:bool)
            n390 = local read "dt"() -> (w739:dbl)
            n391 = case shown="True" w691 {
              tunnel: w673 -> [_ w749]
              tunnel: [w745 w746] -> w686
              tunnel: w690 -> [w745 _]
              frame False {
              }
              frame True {
                n392 = Threshold 1D Array(1:20 ("start index (0)"), 2:0.0 ("threshold y"), 3:w749) -> (0:w746:dbl)
              }
            }
            n393 = Bundle By Name("Y"=w673, "dt"=w739, "t0"=timestamp(0 s since 1904-01-01)) -> (w728:waveform(dbl))  [unwired: 1 in]
            n394 = local read "FF_Wfm"() -> (w727:waveform(dbl))
            n395 = call-poly <vilib>:"Extract Single Tone Information.vi"("time signal in"=w728) -> ("detected amplitude"=w662:dbl, "detected frequency"=→"Freq":dbl)  [unwired: 5 in, 4 out]
            n396 = Subtract(x=w659, y=w662) -> (x-y=w671:dbl)
            n397 = Add(x=w662, y=w659) -> (x+y=w670:dbl)
            n398 = Bundle(w659, w671, w670) -> (→"Slide 8":cluster{dbl, dbl, dbl})  [unwired: 1 in]
            n399 = Build Array(w728, w727) -> (w709:waveform(dbl)[])
            "Waveform Graph 2" <- w709
            n400 = Split 1D Array(array=w673, index=w686) -> (second subarray=w687:dbl[])  [unwired: 1 out]
            n401 = Index Array(array=w709) -> (element #1=w710:waveform(dbl), element #2=w712:waveform(dbl))  [unwired: 2 in]
            n402 = Multiply(x=w662, y=2.0) -> (x*y=w729:dbl)
            "Stroke" <- w729
            "Mean(RAW) Stroke" <- w729
            n403 = local read "Test \nStatus"() -> (w730:bool)
            n404 = Threshold 1D Array(1:180 ("start index (0)"), 2:0.0 ("threshold y"), 3:w687) -> (0:w685:dbl)
            n405 = Unbundle By Name(w710) -> ("Y"=w683:dbl[])
            n406 = Unbundle By Name(w712) -> ("Y"=w684:dbl[])
            n407 = Split 1D Array(array=w684, index=w686) -> (second subarray=w681:dbl[])  [unwired: 1 out]
            n408 = In Range and Coerce(upper limit=1.5, x=w729, lower limit=0.5) -> (In Range?=w733:bool)  [unwired: 1 out]
            n409 = Split 1D Array(array=w687, index=w685) -> (first subarray=w680:dbl[])  [unwired: 1 out]
            n410 = Split 1D Array(array=w681, index=w685) -> (first subarray=w678:dbl[])  [unwired: 1 out]
            n411 = Split 1D Array(array=w683, index="Window") -> (second subarray=w701:dbl[])  [unwired: 1 out]
            n412 = Not(x=w733) -> (.not. x?=w732:bool)
            n413 = And(x=w732, y=w730) -> (x .and. y?=w731:bool)
            n414 = case shown="True" w731 {
              tunnel: [i32[] [] w751] -> _
              frame False {
              }
              frame True {
                n415 = local read "Array"() -> (w754:string[])
                n416 = local read "UnoRead"() -> (w753:string)
                n417 = Build Array (concatenate)(w754, w753) -> (w752:string[])
                "Array" <- w752
                n418 = String Length(string=w752) -> (length=w751:i32[])
              }
            }
            n419 = Array Max & Min(array=w684) -> (max value=w713:dbl, min value=w714:dbl)  [unwired: 2 out]
            n420 = Array Max & Min(array=w701) -> (max value=w715:dbl, min value=w716:dbl)  [unwired: 2 out]
            n421 = call-poly <vilib>:"Hanning Window.vi"("X"=w680) -> ("Windowed X"=w679:dbl[])  [unwired: 1 out]
            n422 = call-poly <vilib>:"Hanning Window.vi"("X"=w678) -> ("Windowed X"=w677:dbl[])  [unwired: 1 out]
            n423 = Subtract(x=w715, y=w716) -> (x-y=w717:dbl)
            n424 = Subtract(x=w713, y=w714) -> (x-y=w718:dbl)
            n425 = Build Array(w679, w677) -> (→"Waveform Graph 4":dbl[][])
            n426 = local read "G_val"() -> (w703:dbl)
            n427 = Divide(x=w718, y=w717) -> (x/y=w706:dbl)
            n428 = call-poly <vilib>:"RMS.vi"("X"=w701) -> ("rms value"=w657:dbl)  [unwired: 1 out]
            "Current (A)" <- w657
            n429 = call-poly <vilib>:"RMS.vi"("X"=w678) -> ("rms value"=w702:dbl)  [unwired: 1 out]
            n430 = local read "Constant (G)"() -> (w695:dbl)
            n431 = Multiply(x=w706, y=0.2) -> (x*y=w708:dbl)
            n432 = Multiply(x=0.8 ("y"), y=w703) -> (x*y=w707:dbl)
            n433 = Divide(x=w702, y=w657) -> (x/y=w696:dbl)
            n434 = Add(x=w708, y=w707) -> (x+y=w675:dbl)
            n435 = Not A Number/Path/Refnum?(number/path/refnum=w675) -> (NaN/Path/Refnum?=w674:bool)
            n436 = Multiply(x=w696, y=0.2) -> (x*y=w697:dbl)
            n437 = Multiply(x=0.8 ("y"), y=w695) -> (x*y=w698:dbl)
            n438 = Select(t=0.0, s=w674, f=w675) -> (s? t:f=w655:dbl)
            "G_val" <- w655
            n439 = Multiply(x=w657, y=w655) -> (x*y=→"Friction Force (N)":dbl)
            n440 = Add(x=w697, y=w698) -> (x+y=w694:dbl)
            "Constant (G)" <- w694
            n441 = Bundle(w694, "t"=w655) -> (→"pk-pk":cluster{dbl, "t":dbl})  [unwired: 1 in]
          }
          frame #4 {
            # "C:\\WinDucom\\data\\"
            # "?C:\\LAB-IQ-NXT\\data"
            n442 = case shown="True" "save dpt" {
              frame False {
              }
              frame True {
                n443 = local read "FF buffer"() -> (w773:dbl[])
                n444 = local read "ABS DP"() -> (w772:dbl[])
                n445 = Build Array(w773, w772) -> (w768:dbl[][])
                n446 = Transpose 2D Array(2D array=w768) -> (transposed array=w767:dbl[][])
                n447 = Array To Spreadsheet String(delimiter (Tab)=";", array=w767, 3:"" ("format string")) -> (spreadsheet string=w769:string)
                "String 9" <- w769
